vi "CI Project Builder.vi"() -> ()   [LabVIEW 2014]
uses:
  LabVIEW Tool/Actors/Project Builder/Project Builder.lvclass
  <vilib>/ActorFramework/Actor/Actor.lvclass
panel:
  out "error out":errorcluster
  # "LabVIEW CI Project Builder"
  # "Version 1.0"
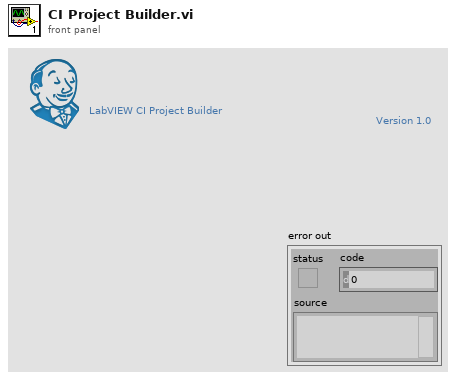
[diagram p1: front panel]
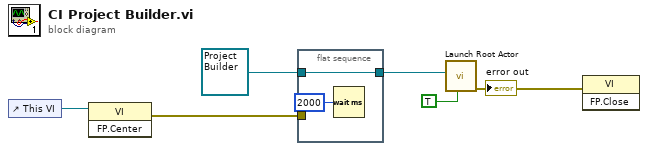
[diagram p0: block diagram]
diagram:
  n1 = control-ref of="This VI"() -> (w1:refnum<vi>)
  n2 = invoke class="VI" method="FP.Center"(reference=w1) -> (error out=w2:errorcluster)  [unwired: 2 in, 2 out]
  n3 = flat-sequence {
    tunnel: refnum<class "Project Builder.lvclass"> refnum ("Project Builder.lvclass") -> [w8]
    tunnel: [w8] -> w4
    tunnel: w2 -> [_]
    frame #0 {
      n4 = Wait (ms)(milliseconds to wait=u32 2000) -> ()  [unwired: 1 out]
    }
  }
  n5 = call <vilib>:"Launch Root Actor.vi"("Open Actor Core front panel? (F)"=TRUE, "Actor"=w4) -> ("error out"=w3:errorcluster)  [unwired: 8 in, 1 out]
  "error out" <- w3
  n6 = invoke class="VI" method="FP.Close"(error in=w3) -> ()  [unwired: 2 in, 3 out]
